vi "4) (b) Sub VI (Temperature Conversion).vi"(8 "Boolean":bool, 11 "Temperature (F)":dbl) -> (3 "Numeric":dbl)   [LabVIEW 2018]
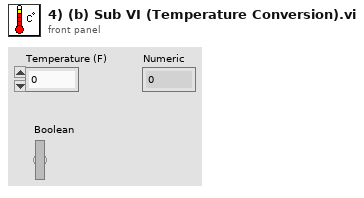
[diagram p1: front panel]
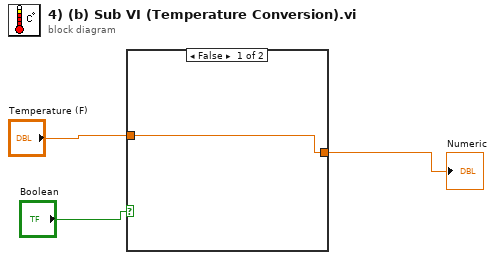
[diagram p0: block diagram]
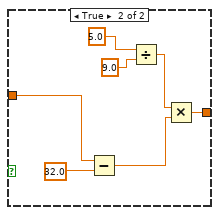
[diagram p2: hidden frame]
diagram:
  n1 = case shown="False" "Boolean" {
    tunnel: "Temperature (F)" -> [w4 w9]
    tunnel: [w4 w7] -> w2
    frame False {
    }
    frame True {
      n2 = Subtract(x=w9, y=32.0 ("x-y")) -> (x-y=w6:dbl)
      n3 = Divide(x=5.0 ("x/y"), y=9.0) -> (x/y=w5:dbl)
      n4 = Multiply(x=w5, y=w6) -> (x*y=w7:dbl)
    }
  }
  "Numeric" <- w2
